vi "n set standby list.vi"(8 "error in (no error)":errorcluster, 9 "pulse":u16, 10 "half_period":u16, 11 "n":u16) -> (0 "error out":errorcluster)   [LabVIEW 2015, in "SCANalone4x64.lvlib"]
doc: "__declspec(dllimport) void __stdcall n_set_standby_list(unsigned short n, unsigned short half_period, unsigned short pulse);"
uses:
  <userlib>/SCANalone4x64/SCANalone4x64.lvlib
  <userlib>/SCANalone4x64/SCANalone4x64.dll
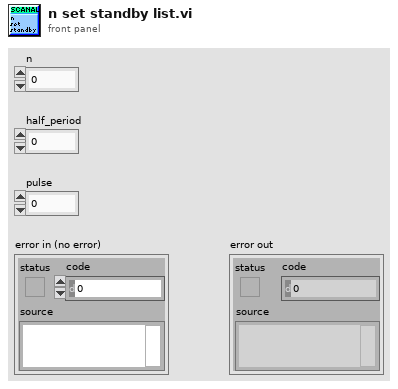
[diagram p1: front panel]
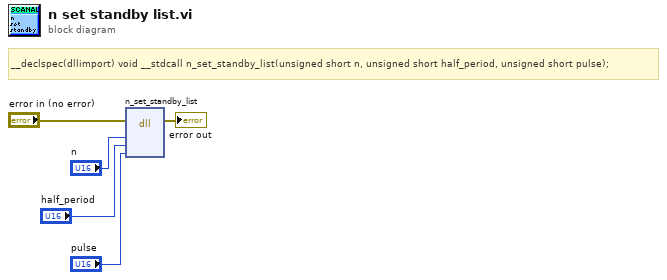
[diagram p0: block diagram]
diagram:
  # "__declspec(dllimport) void __stdcall n_set_standby_list(unsigned short n, unsigned short half_period, unsigned short pulse);"
  n1 = dll-call lib="C:/Program Files/National Instruments/LabVIEW 2015/user.lib/SCANalone4x64/SCANalone4x64.*" fn="n_set_standby_list"(error in="error in (no error)", "n"="n", "half_period"="half_period", "pulse"="pulse") -> (error out=→"error out":errorcluster)  [unwired: 6 in, 1 out]
